vi "Build Folder Config.vi"(11 "Library":refnum<vi>) -> (3 "Folders":T1[](array[typedef]))   [LabVIEW 2020, in "Negentropic IDE.lvlib"]
uses:
  <resource>/Framework/Providers/Negentropic IDE/Negentropic IDE/Negentropic IDE.lvlib
  <resource>/Framework/Providers/Negentropic IDE/Negentropic IDE/Folder Config.ctl
  <resource>/Framework/Providers/Negentropic IDE/Negentropic IDE/Scope.ctl
  <resource>/Framework/Providers/Negentropic IDE/Negentropic IDE/Folder Enumeration Item.ctl
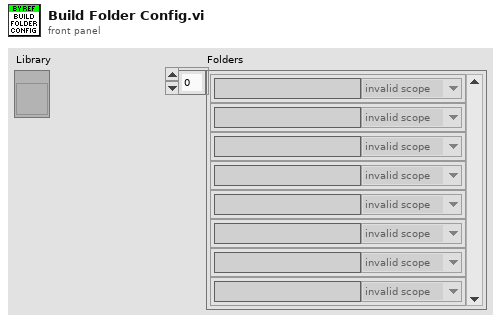
[diagram p1: front panel]
types:
  T1 = typedef "Negentropic IDE.lvlib/Folder Config.ctl" = cluster{"Path":string, "Scope":T2}
  T2 = typedef "Negentropic IDE.lvlib/Scope.ctl" = enum32{"invalid scope", "public", "private", "protected", "community"}
  T3 = typedef "Negentropic IDE.lvlib/Folder Enumeration Item.ctl" = cluster{"Path":string, "Refnum":refnum<vi>, "Virtual Folder":bool, "Scope":T2}
  T4 = enum32{"invalid scope", "public", "private", "protected", "community"}
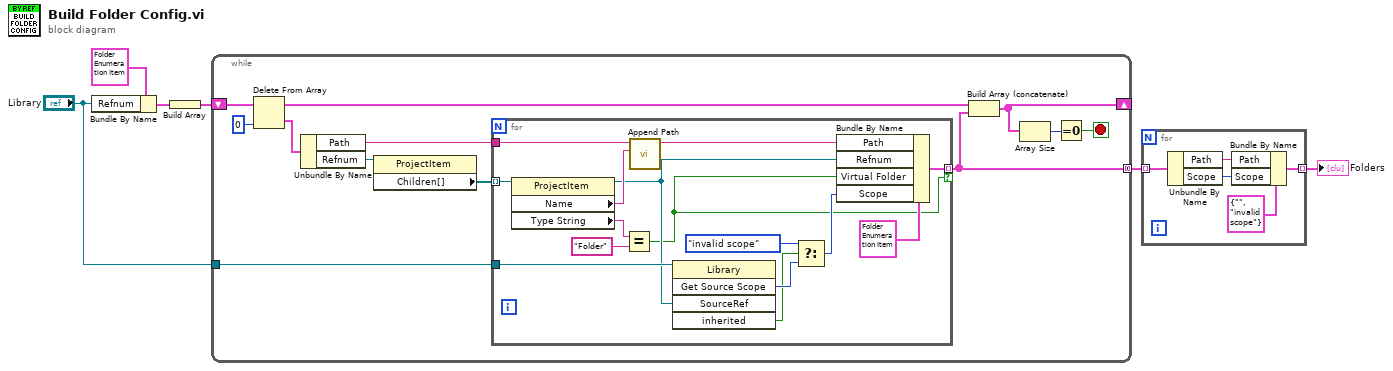
[diagram p0: block diagram]
diagram:
  n1 = Bundle By Name(cluster=T3 {"Path"="", "Refnum"=refnum, "Virtual Folder"=FALSE, "Scope"=enum."invalid scope"} ("Folder Enumeration Item"), "Refnum"="Library") -> (w5:T3)
  n2 = Build Array(w5) -> (w4:T3[])
  n3 = while {
    shift-right: [w10] -> _
    shift-left: w4 -> [w18]
    tunnel: "Library" -> [w12]
    tunnel: [w7] -> w2 mode=concatenating
    stop <- w8 stop-if-true
    n4 = Delete From Array(array=w18, index=0) -> (deleted portion=w16:T3, array with subset deleted=w11:T3[])  [unwired: 1 in]
    n5 = Unbundle By Name(w16) -> ("Path"=w13:string, "Refnum"=w15:refnum<vi>)
    n6 = property class="ProjectItem"(reference=w15) -> ("Children[]"=w14:refnum<vi>[])  [unwired: 1 in, 2 out]
    n7 = for {
      tunnel: w14 -> [w32] mode=indexing
      tunnel: w13 -> [w33]
      tunnel: w12 -> [w26]
      tunnel: [w20] -> w7 mode=indexing if=w19
      n8 = property class="ProjectItem"(reference=w32) -> (reference out=w25:refnum<vi>, "Name"=w31:string, "Type String"=w30:string)  [unwired: 1 in, 1 out]
      n9 = Equal?(x=w30, y="Folder") -> (x = y?=w19:bool)
      n10 = call <resource>:"Append Path.vi"("Item Name"=w31, "Parent Path"=w33) -> ("Path"=w27:string)  [unwired: 9 in]
      n11 = invoke class="Library" method="Get Source Scope"(reference=w26, "SourceRef"=w25) -> ("GetSourceScope"=w24:T4, "inherited"=w23:bool)  [unwired: 3 in, 3 out]
      n12 = Select(t=T4."invalid scope", s=w23, f=w24) -> (s? t:f=w21:T4)
      n13 = Bundle By Name(cluster=T3 {"Path"="", "Refnum"=refnum, "Virtual Folder"=FALSE, "Scope"=enum."invalid scope"} ("Folder Enumeration Item"), "Path"=w27, "Refnum"=w25, "Virtual Folder"=w19, "Scope"=w21) -> (w20:T3)
    }
    n14 = Build Array (concatenate)(w11, w7) -> (w10:T3[])
    n15 = Array Size(array=w10) -> (size(s)=w9:i32)
    n16 = Equal To 0?(x=w9) -> (x = 0?=w8:bool)
  }
  n17 = for {
    tunnel: w2 -> [w38] mode=indexing
    tunnel: [w34] -> w1 mode=indexing
    n18 = Unbundle By Name(w38) -> ("Path"=w36:string, "Scope"=w35:T2)
    n19 = Bundle By Name(cluster=T1 {"Path"="", "Scope"=enum."invalid scope"} ("Folder Config"), "Path"=w36, "Scope"=w35) -> (w34:T1)
  }
  "Folders" <- w1
